vi "createStreamingDataAlgorithm.vi"(8 "error in (no error)":errorcluster, 10 "Stream Mode Algorithm":T1, 11 "SDAFactory in":refnum<class "SDAFactory.lvclass">) -> (0 "error out":errorcluster, 2 "StreamingDataAlgorithm":refnum<class "StreamingDataAlgorithm.lvclass">, 3 "SDAFactory out":refnum<class "SDAFactory.lvclass">)   [LabVIEW 2013, in "SDAFactory.lvclass"]
uses:
  SDAFactory.lvclass
  StreamingDataAlgorithm/StreamingDataAlgorithm.lvclass
  Configuration/Stream Mode Algorithm.ctl
  StreamingDataAlgorithms/FrontPanelValuesSimple/FrontPanelValuesSimple.lvclass
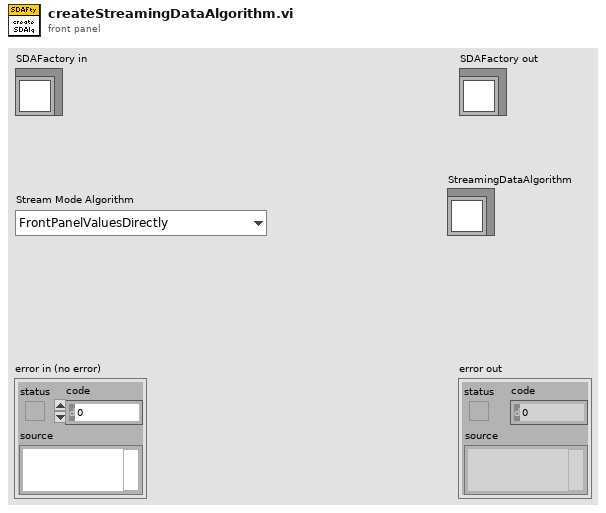
[diagram p1: front panel]
types:
  T1 = typedef "Stream Mode Algorithm.ctl" = enum16{"FrontPanelValuesDirectly"}
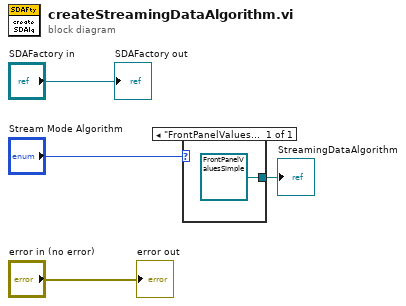
[diagram p0: block diagram]
diagram:
  n1 = case shown="\"FrontPanelValuesDirectly\"" "Stream Mode Algorithm" {
    tunnel: [refnum<class "FrontPanelValuesSimple.lvclass"> refnum ("FrontPanelValuesSimple.lvclass")] -> w1
    frame "FrontPanelValuesDirectly" {
    }
  }
  "StreamingDataAlgorithm" <- w1
  "error out" <- "error in (no error)"
  "SDAFactory out" <- "SDAFactory in"
